vi "Auto Indicator.vi"() -> ()   [LabVIEW 2014]
uses:
  Global Var.vi
panel:
  out "Default State":T1
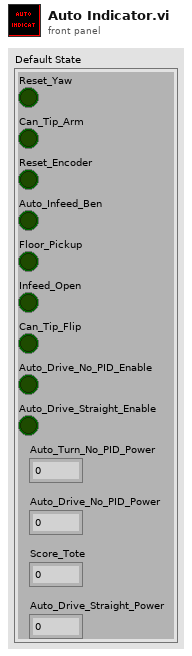
[diagram p1: front panel]
types:
  T1 = cluster{"Reset_Yaw":bool, "Can_Tip_Arm":bool, "Reset_Encoder":bool, "Auto_Infeed_Ben":bool, "Floor_Pickup":bool, "Infeed_Open":bool, "Can_Tip_Flip":bool, "Auto_Drive_No_PID_Enable":bool, "Auto_Drive_Straight_Enable":bool, "Auto_Turn_No_PID_Power":dbl, "Auto_Drive_No_PID_Power":dbl, "Score_Tote":dbl, "Auto_Drive_Straight_Power":dbl}
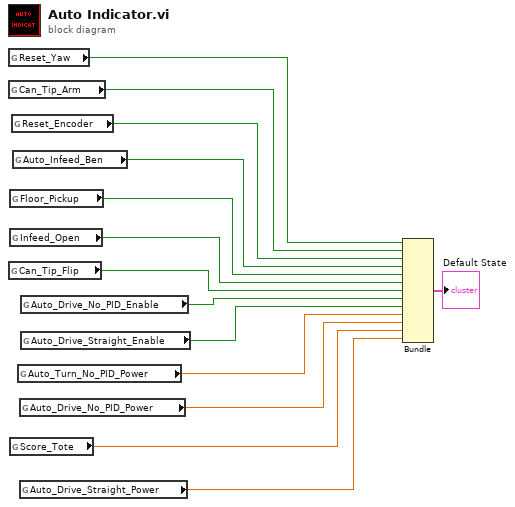
[diagram p0: block diagram]
diagram:
  n1 = global read "Global Var.vi" "Reset_Yaw"() -> (w14:bool)
  n2 = global read "Global Var.vi" "Can_Tip_Arm"() -> (w13:bool)
  n3 = global read "Global Var.vi" "Can_Tip_Flip"() -> (w8:bool)
  n4 = global read "Global Var.vi" "Floor_Pickup"() -> (w10:bool)
  n5 = global read "Global Var.vi" "Infeed_Open"() -> (w9:bool)
  n6 = global read "Global Var.vi" "Score_Tote"() -> (w3:dbl)
  n7 = global read "Global Var.vi" "Reset_Encoder"() -> (w12:bool)
  n8 = global read "Global Var.vi" "Auto_Infeed_Ben"() -> (w11:bool)
  n9 = global read "Global Var.vi" "Auto_Turn_No_PID_Power"() -> (w5:dbl)
  n10 = global read "Global Var.vi" "Auto_Drive_No_PID_Power"() -> (w4:dbl)
  n11 = global read "Global Var.vi" "Auto_Drive_Straight_Power"() -> (w2:dbl)
  n12 = global read "Global Var.vi" "Auto_Drive_No_PID_Enable"() -> (w7:bool)
  n13 = global read "Global Var.vi" "Auto_Drive_Straight_Enable"() -> (w6:bool)
  n14 = Bundle("Reset_Yaw"=w14, "Can_Tip_Arm"=w13, "Reset_Encoder"=w12, "Auto_Infeed_Ben"=w11, "Floor_Pickup"=w10, "Infeed_Open"=w9, "Can_Tip_Flip"=w8, "Auto_Drive_No_PID_Enable"=w7, "Auto_Drive_Straight_Enable"=w6, "Auto_Turn_No_PID_Power"=w5, "Auto_Drive_No_PID_Power"=w4, "Score_Tote"=w3, "Auto_Drive_Straight_Power"=w2) -> (→"Default State":T1)  [unwired: 1 in]
